vi "2 Global.vi"() -> ()   [LabVIEW 2011]
uses:
  2 Typedefs/UTM Location.ctl
  2 Typedefs/apparent wind.ctl
  2 Typedefs/apparent wind speed.ctl
  2 Typedefs/apparent wind direction.ctl
  2 Typedefs/robot velocity.ctl
  2 Typedefs/heading.ctl
  2 Typedefs/generalized actuator status.ctl
  2 Typedefs/indicator LED.ctl
  2 Typedefs/generalized sensor status.ctl
  2 Typedefs/Which Boat.ctl
  0x2-OCU-Think Comm/0x2 Typedefs/manual override.ctl
  2 Typedefs/setpoints to boat.ctl
  2 Typedefs/sail setpt.ctl
  2 Typedefs/rudder angle.ctl
  2 Typedefs/Velocity.ctl
  2 Typedefs/rate of turn.ctl
  2 Typedefs/absolute wind direction.ctl
  2 Typedefs/absolute wind speed.ctl
  2 Typedefs/pitch and roll.ctl
  0x2-OCU-Think Comm/0x2 Typedefs/Waypoints List.ctl
  2 Classes/Waypoint/Waypoint.lvclass
  0x2-OCU-Think Comm/0x2 Typedefs/Current Waypoint.ctl
  2 Classes/Missions/GenericMission/GenericMission.lvclass
  2 Typedefs/Goodness Fns Indicator.ctl
  2 Typedefs/UTM Circle.ctl
panel:
  in  "E-Stop":bool
  in  "Globals":T1(tab)
  out "Don't Tip?":bool
  out "Network \nfreq.":dbl
  out "E-stop freq.":dbl
  out "Act freq.":dbl
  out "Sense freq.":dbl
  out "Think freq.":dbl
  in  "Which Boat Am I?":T2
  out "Sensor Status":T3={"Sensor Connected"=FALSE, "Sensor Initialized"=FALSE, "Sensor OK"=FALSE, "Latest Error String"="Serial port probably timed out. Source: VISA Read in 1A Read Sensor Data.vi->Main.vi", "GPS Lock"=FALSE}
  out "Sail Actuator Status":T5
  out "Rudder Actuator Status":T5
  in  "Battery Voltage":dbl
  out "Estimated Error":dbl
  in  "Robot Pitch/Roll":T6 {"Roll" format="%05.1f"; "Pitch" format="%05.1f"}
  in  "Robot\nRate of Turn":T7 format="%05.1f"
  in  "Robot\nHeading":T8 format="%05.1f"
  in  "Robot UTM Location":T9 {"North" format="%#_10f"; "East" format="%#_8f"}
  in  "Robot Velocity":T10
  out "Overview Image":T11(plugin-control)
  in  "Defilter Wind Data":bool=TRUE
  in  "Shift Goal for Currents":bool
  in  "Let Sail Out on Windcross":bool
  in  "Crossing the Wind":bool
  in  "RP Autonomous":bool
  in  "RP Speed ABS":T12
  in  "RP Direction ABS":T13
  in  "RP Direction":T14
  in  "RP Speed":T15
  in  "Runprotection":bool
  in  "Absolute Water Current Vector":T16 {"East" format="%#_5g"}
  in  "Absolute Wind\nSpeed":T12
  in  "Absolute Wind\nDirection (º)":T13
  in  "Absolute Wind":T16 {"East" format="%#_5g"}
  in  "Apparent Wind\nDirection (º)":T14
  in  "Apparent Wind\nSpeed":T15
  in  "Apparent Wind":T17
  in  "Round Buoy Safety":dbl
  in  "Shifted Waypoint":refnum<class "Waypoint.lvclass">
  out "Current Mission":refnum<class "GenericMission.lvclass">
  in  "Current Waypoint":T18
  in  "Waypoints Array":T19
  in  "Manual Override Cluster":T20
  in  "Sail Position":T22
  in  "Rudder Angle":T23
  out "Goodness Functions":T24
  in  "Global No Sail Circles":T25[](array[typedef])
  in  "Setpoints to boat":T21
  out "Optimal Heading":dbl
  # "All distances in meters, all speeds in meters per second\nAll angles in degrees, clockwise with 0 being positive North if in global reference frame or 0 being Fore in boat ref frame.\nX-Y make a right handed coordinate system with Z pointing up\nPositive Rudder angle makes the boat turn right\nLocation Coordinates are in UTM format"
  # "Loop Rates"
  # "As Measured"
  # "As Calculated"
  # "As Measured"
  # "As Calculated"
  # "From Planning Functions"
  # "Path Planning"
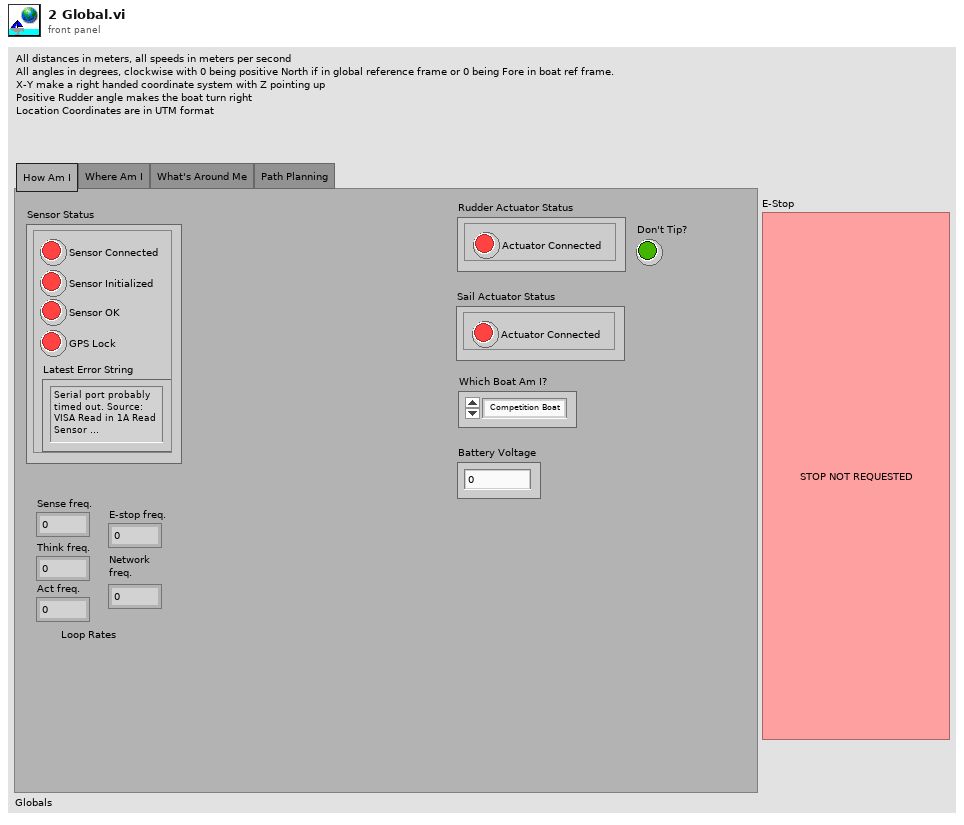
[diagram p1: front panel]
types:
  T1 = enum32{"How Am I", "Where Am I", "What's Around Me", "Path Planning"}
  T2 = typedef "Which Boat.ctl" = enum16{"Competition Boat", "Small RC", "Simulation"}
  T3 = typedef "generalized sensor status.ctl" = cluster{"Sensor Connected":T4, "Sensor Initialized":T4, "Sensor OK":T4, "Latest Error String":string, "GPS Lock":T4}
  T4 = typedef "indicator LED.ctl" = bool
  T5 = typedef "generalized actuator status.ctl" = cluster{"Actuator Connected":T4}
  T6 = typedef "pitch and roll.ctl" = cluster{"Pitch":dbl, "Roll":dbl}
  T7 = typedef "rate of turn.ctl" = dbl
  T8 = typedef "heading.ctl" = dbl
  T9 = typedef "UTM Location.ctl" = cluster{"UTM Zone":dbl, "Hemisphere":enum16{"North", "South"}, "East":dbl, "North":dbl}
  T10 = typedef "robot velocity.ctl" = cluster{"East":dbl, "North":dbl}
  T11 = typedef "IMAQ Image.ctl" = refnum<image>
  T12 = typedef "absolute wind speed.ctl" = dbl
  T13 = typedef "absolute wind direction.ctl" = dbl
  T14 = typedef "apparent wind direction.ctl" = dbl
  T15 = typedef "apparent wind speed.ctl" = dbl
  T16 = typedef "Velocity.ctl" = cluster{"East":dbl, "North":dbl}
  T17 = typedef "apparent wind.ctl" = cluster{"Toward Fore":dbl, "Toward Starboard":dbl}
  T18 = typedef "Current Waypoint.ctl" = i32
  T19 = typedef "Waypoints List.ctl" = refnum<class "Waypoint.lvclass">[]
  T20 = typedef "manual override.ctl" = cluster{"Override Active Rudder":bool, "Setpoints":T21, "Override Active Sail":bool}
  T21 = typedef "setpoints to boat.ctl" = cluster{"Sail Position":T22, "Rudder Angle":T23}
  T22 = typedef "sail setpt.ctl" = dbl
  T23 = typedef "rudder angle.ctl" = dbl
  T24 = typedef "Goodness Fns Indicator.ctl" = cluster{dbl, dbl, dbl[][]}
  T25 = typedef "UTM Circle.ctl" = cluster{"UTM Zone":dbl, "Hemisphere":enum16{"North", "South"}, "East":dbl, "North":dbl, "Radius":dbl}
diagram:
